vi "HelpOn.vi"(8 "Error In":errorcluster, 11 "reference in":refnum<class "Wolfram.lvclass">) -> (0 "Error Out":errorcluster, 3 "reference out":refnum<class "Wolfram.lvclass">)   [LabVIEW 2020, in "Wolfram.lvclass"]
uses:
  Wolfram.lvclass
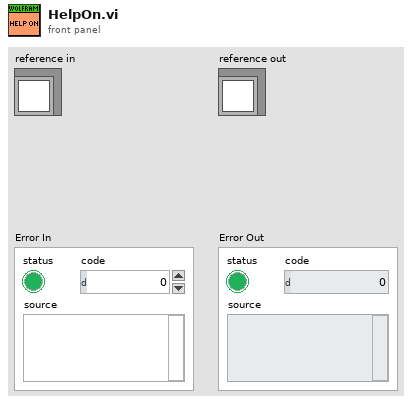
[diagram p1: front panel]
types:
  T1 = typedef "Wolfram.lvclass/ObjectAttributes.ctl" = cluster{"AnswerRef":refnum<vi>}
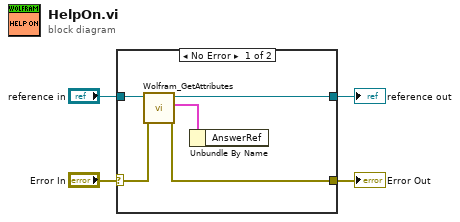
[diagram p0: block diagram]
diagram:
  n1 = case shown="No Error" "Error In" {
    selector: "Error In" -> [w9 w11]
    tunnel: [w7 w11] -> w3
    tunnel: [w5 w10] -> w1
    tunnel: "reference in" -> [w6 w10]
    frame No Error {
      n2 = call "Wolfram_GetAttributes.vi"("error in (no error)"=w9, "reference in"=w6) -> ("error out"=w7:errorcluster, "Data"=w8:T1, "reference out"=w5:refnum<class "Wolfram.lvclass">)  [unwired: 6 in, 1 out]
      n3 = Unbundle By Name(w8) -> ()  [unwired: 1 out]
    }
    frame Error {
    }
  }
  "Error Out" <- w3
  "reference out" <- w1
